vi "ALTS-2015 Startup.vi"() -> ()   [LabVIEW 2013]
uses:
  Controls/ALTS-2015 LV2GBL Restart Options.ctl
panel:
  out "Status":string
  out "Error Out":errorcluster
  in  "Error In":errorcluster
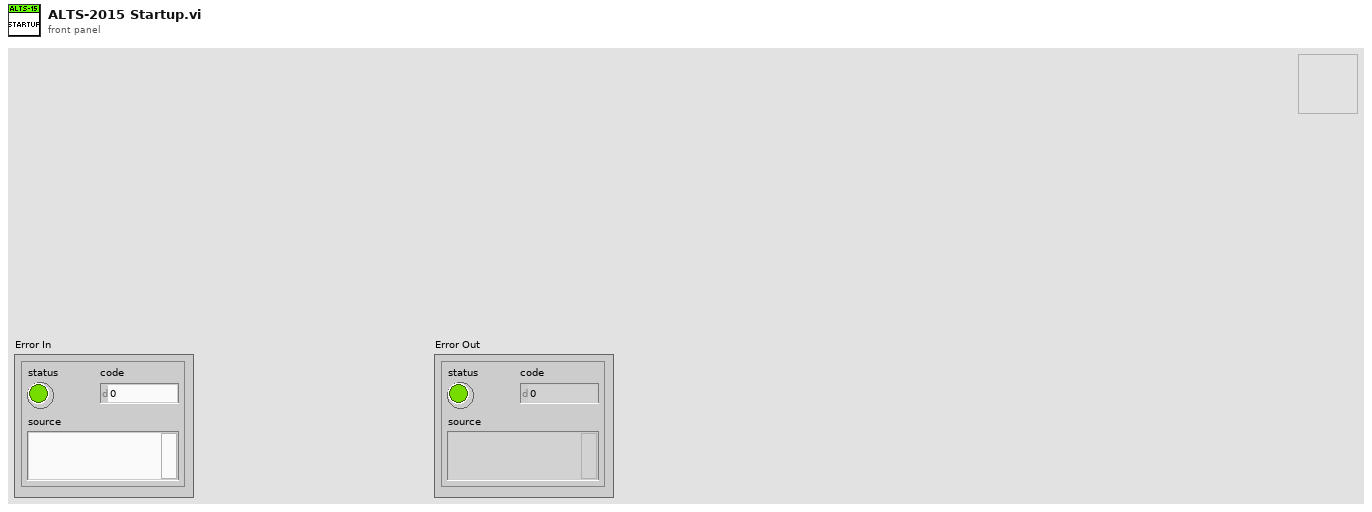
[diagram p1: front panel]
types:
  T1 = typedef "ALTS-2015 LV2GBL Restart Options.ctl" = enum16{"Get All Data", "Set Restart Notifier Ref", "Store Authentication Data"}
  T2 = enum32{"Invalid", "Standard", "Closed", "Hidden", "Minimized", "Maximized"}
  T3 = enum32{"Bad", "Idle", "Run top level", "Running"}
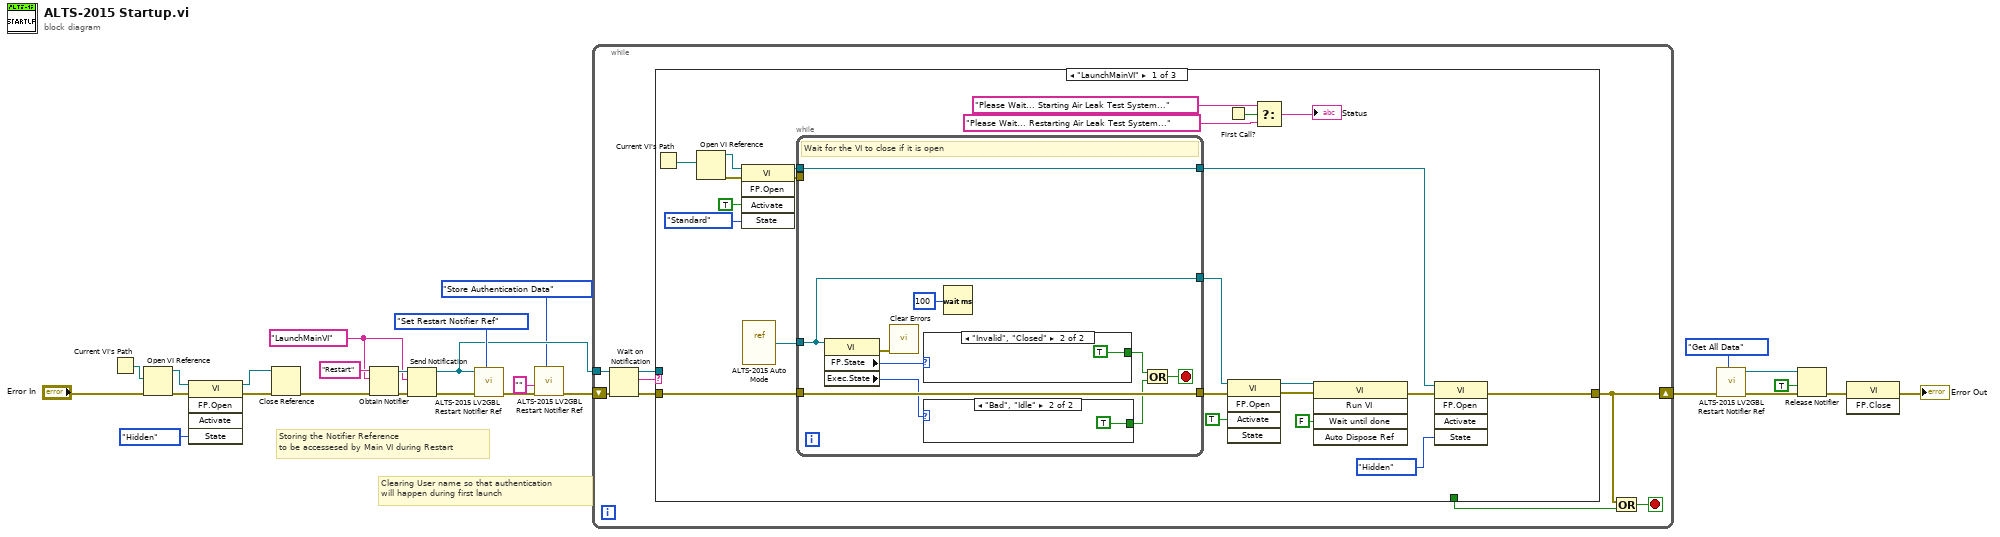
[diagram p0: block diagram]
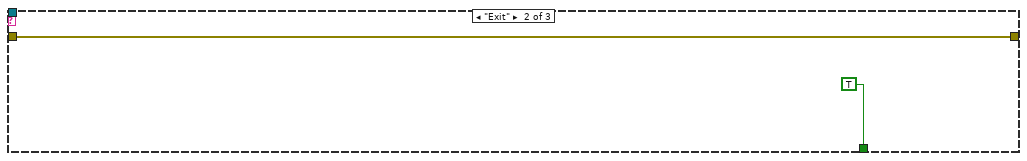
[diagram p4: hidden frame]
diagram:
  w8 = "LaunchMainVI"
  # "Clearing User name so that authentication \nwill happen during first launch"
  # "Storing the Notifier Reference\nto be accessesed by Main VI during Restart"
  n1 = Current VI's Path() -> (path=w18:path)
  n2 = Open VI Reference(vi path=w18, error in (no error)="Error In") -> (vi reference=w22:refnum<vi>, error out=w23:errorcluster)  [unwired: 4 in]
  n3 = invoke class="VI" method="FP.Open"(reference=w22, error in=w23, "State"=T2."Hidden") -> (reference out=w14:refnum<vi>, error out=w13:errorcluster)  [unwired: 2 in, 3 out]
  n4 = Close Reference(reference=w14, error in (no error)=w13) -> (error out=w20:errorcluster)
  n5 = Obtain Notifier(name (unnamed)="Restart", notification data type=w8, error in (no error)=w20) -> (notifier out=w26:refnum<notifier>, error out=w25:errorcluster)  [unwired: 1 in, 1 out]
  n6 = Send Notification(notification=w8, notifier=w26, error in (no error)=w25) -> (notifier out=w6:refnum<notifier>, error out=w11:errorcluster)
  n7 = call "ALTS-2015 LV2GBL Restart Notifier Ref.vi"("Options"=ALTS-2015_LV2GBL_Restart_Options."Set Restart Notifier Ref", "Error In"=w11, "Restart Notifier In"=w6) -> ("Error Out"=w5:errorcluster)  [unwired: 6 in, 2 out]
  n8 = call "ALTS-2015 LV2GBL Restart Notifier Ref.vi"("Options"=ALTS-2015_LV2GBL_Restart_Options."Store Authentication Data", "Error In"=w5, "Authenticated User Name"="") -> ("Error Out"=w4:errorcluster)  [unwired: 6 in, 2 out]
  n9 = while {
    shift-right: [w28] -> w17
    shift-left: w4 -> [w34]
    tunnel: w6 -> [w30]
    stop <- w27 stop-if-true
    n10 = Wait on Notification(notifier=w30, error in (no error)=w34) -> (notifier out=w31:refnum<notifier>, notification=w33:string, error out=w32:errorcluster)  [unwired: 2 in, 1 out]
    n11 = case shown="\"LaunchMainVI\"" w33 {
      tunnel: [w44 w70 w72] -> w28
      tunnel: w32 -> [w57 w70 w72]
      tunnel: w31 -> [_ _ _]
      tunnel: [_ TRUE _] -> w29
      frame "LaunchMainVI" {
        n12 = Current VI's Path() -> (path=w52:path)
        n13 = Open VI Reference(vi path=w52) -> (vi reference=w53:refnum<vi>, error out=w51:errorcluster)  [unwired: 5 in]
        n14 = invoke class="VI" method="FP.Open"(reference=w53, error in=w51, "Activate"=TRUE ("Activate?"), "State"=T2."Standard") -> (reference out=w49:refnum<vi>, error out=w48:errorcluster)  [unwired: 1 in, 3 out]
        n15 = vi-ref "ALTS-2015 Auto Mode.vi"() -> (w56:refnum<vi>)
        n16 = while {
          tunnel: w57 -> [w63]
          tunnel: w56 -> [w64]
          tunnel: [w64] -> w40
          tunnel: [w63] -> w43
          tunnel: w49 -> [w62]
          tunnel: w48 -> [_]
          tunnel: [w62] -> w46
          stop <- w58 stop-if-true
          # "Wait for the VI to close if it is open"
          n17 = property class="VI"(reference=w64) -> (error out=w66:errorcluster, "FP.State"=w67:T2, "Exec.State"=w60:T3)  [unwired: 1 in, 1 out]
          n18 = call <vilib>:"Clear Errors.vi"("error in (no error)"=w66) -> ()  [unwired: 6 in, 1 out]
          n19 = case shown="\"Invalid\", \"Closed\"" w67 {
            tunnel: [_ TRUE] -> w61
            frame "Standard", Default {
            }
            frame "Invalid", "Closed" {
            }
          }
          n20 = case shown="\"Bad\", \"Idle\"" w60 {
            tunnel: [_ TRUE] -> w59
            frame Default {
            }
            frame "Bad", "Idle" {
            }
          }
          n21 = Wait (ms)(milliseconds to wait=u32 100) -> ()  [unwired: 1 out]
          n22 = Or(x=w61, y=w59) -> (x .or. y?=w58:bool)
        }
        n23 = First Call?() -> (First Call?: T/F=w38:bool)
        n24 = invoke class="VI" method="FP.Open"(reference=w40, error in=w43, "Activate"=TRUE ("Activate?")) -> (reference out=w39:refnum<vi>, error out=w42:errorcluster)  [unwired: 2 in, 3 out]
        n25 = Select(t="Please Wait... Starting Air Leak Test System..." ("Status"), s=w38, f="Please Wait... Restarting Air Leak Test System..." ("Status")) -> (s? t:f=→"Status":string)
        n26 = invoke class="VI" method="Run VI"(reference=w39, error in=w42, "Wait until done"=FALSE ("Wait Until Done")) -> (error out=w45:errorcluster)  [unwired: 2 in, 4 out]
        n27 = invoke class="VI" method="FP.Open"(reference=w46, error in=w45, "State"=T2."Hidden") -> (error out=w44:errorcluster)  [unwired: 2 in, 4 out]
      }
      frame "Exit" {
      }
      frame Default {
        # "Will Never Happen"
      }
    }
    n28 = Or(x=w28, y=w29) -> (x .or. y?=w27:bool)
  }
  n29 = call "ALTS-2015 LV2GBL Restart Notifier Ref.vi"("Options"=ALTS-2015_LV2GBL_Restart_Options."Get All Data", "Error In"=w17) -> ("Error Out"=w10:errorcluster, "Restart Notifier Out"=w9:refnum<notifier>)  [unwired: 7 in, 1 out]
  n30 = Release Notifier(notifier=w9, force destroy? (F)=TRUE, error in (no error)=w10) -> (error out=w16:errorcluster)  [unwired: 2 out]
  n31 = invoke class="VI" method="FP.Close"(error in=w16) -> (error out=→"Error Out":errorcluster)  [unwired: 2 in, 2 out]
